vi "CAN-LIN Raw Bus Capture TS Client.vi"(11 "Client":string) -> (0 "error out":errorcluster)   [LabVIEW 2025]
uses:
  can-lin/CAN-LIN Raw Bus Capture UI/OOB gRPC Client/RPC Messages/hwval_GenericRequest.ctl
  can-lin/CAN-LIN Raw Bus Capture UI/OOB gRPC Client/OOB gRPC Client.lvlib
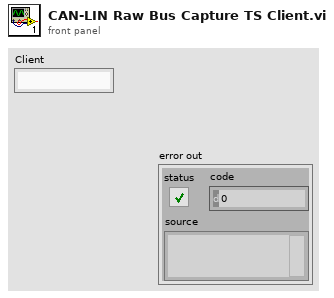
[diagram p1: front panel]
types:
  T1 = typedef "grpc-lvsupport-release.lvlib/grpcId.ctl" = u64
  T2 = typedef "OOB gRPC Client.lvlib/hwval_GenericRequest.ctl" = cluster{"Command":string, "Payload":u8[]}
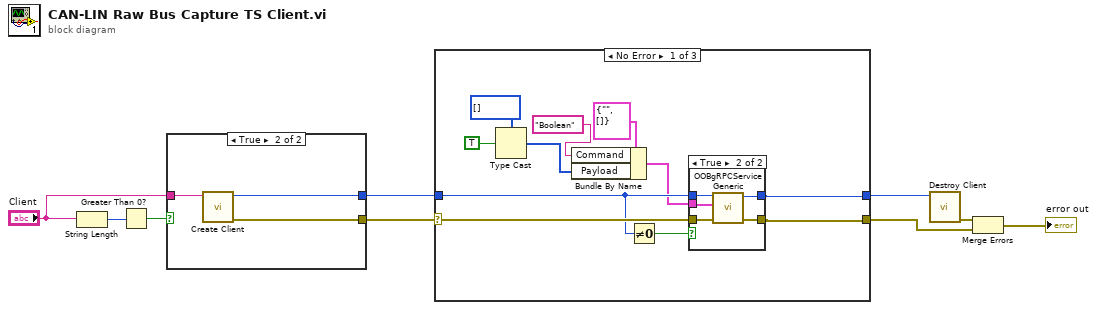
[diagram p0: block diagram]
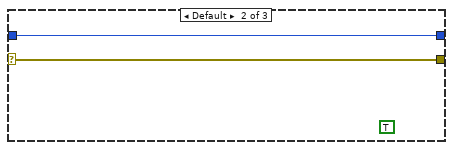
[diagram p3: hidden frame]
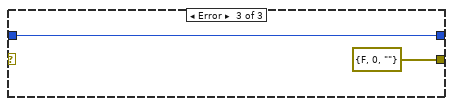
[diagram p4: hidden frame]
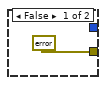
[diagram p5: hidden frame]
diagram:
  n1 = String Length(string="Client") -> (length=w3:i32)
  n2 = Greater Than 0?(x=w3) -> (x > 0?=w2:bool)
  n3 = case shown="True" w2 {
    tunnel: [_ w13] -> w9
    tunnel: [errorcluster {"status"=TRUE, "code"=-1, "source"="Set  a valid Server Port"} ("error out") w12] -> w8
    tunnel: "Client" -> [_ w11]
    frame False {
    }
    frame True {
      n4 = call "Create Client.vi"("address"=w11) -> ("error out"=w12:errorcluster, "gRPC ID Out"=w13:T1)  [unwired: 9 in]
    }
  }
  n5 = case shown="No Error" w8 {
    selector: w8 -> [w24 w32 _]
    tunnel: [w15 w32 errorcluster {"status"=FALSE, "code"=0, "source"=""} ("error IO")] -> w6
    tunnel: w9 -> [w23 w33 w34]
    tunnel: [w14 w33 w34] -> w7
    frame No Error {
      n6 = Type Cast(type=u8[] [] ("Payload"), x=TRUE ("STOP")) -> (*(type *) &x=w18:u8[])
      n7 = Bundle By Name(cluster=T2 {"Command"="", "Payload"=[]} ("Request Data"), "Command"="Boolean", "Payload"=w18) -> (w22:T2)
      n8 = Not Equal To 0?(x=w23) -> (x != 0?=w21:bool)
      n9 = case shown="True" w21 {
        tunnel: [w26 w30] -> w14
        tunnel: [w25 w29] -> w15
        tunnel: w23 -> [w26 w31]
        tunnel: w24 -> [w25 w28]
        tunnel: w22 -> [_ w27]
        frame False {
        }
        frame True {
          n10 = call "OOBgRPCService Generic.vi"("error in"=w28, "Request Data"=w27, "gRPC ID"=w31) -> ("error out"=w29:errorcluster, "gRPC ID out"=w30:T1)  [unwired: 6 in, 1 out]
        }
      }
    }
    frame Default {
      (unwired) TRUE
    }
    frame Error {
    }
  }
  n11 = call "Destroy Client.vi"("gRPC ID"=w7) -> ("error out"=w4:errorcluster)  [unwired: 10 in]
  n12 = Merge Errors(w4, w6) -> (→"error out":errorcluster)
